vi "DW2BA(glue).vi"(10 "DW01":i16, 11 "DW00":i16) -> (2 "秒數":dbl)   [LabVIEW 2019]
panel:
  out "翻轉後接起再翻轉":u32
  out "翻轉後接起":u32
  out "無翻轉接起後翻轉":u32
  out "無翻轉直接接起來":i32
  out "翻轉後接起再翻轉":bool[](array[boolean])
  out "無翻轉接起後翻轉":bool[](array[boolean])
  out "翻轉後接起":bool[](array[boolean])
  out "無翻轉直接接起來":bool[](array[boolean])
  out "DW01":bool[](array[boolean])
  out "DW00":bool[](array[boolean])
  # "一共有八種可能:\n這邊是DW01+DW00\n另一種是DW00+DW01"
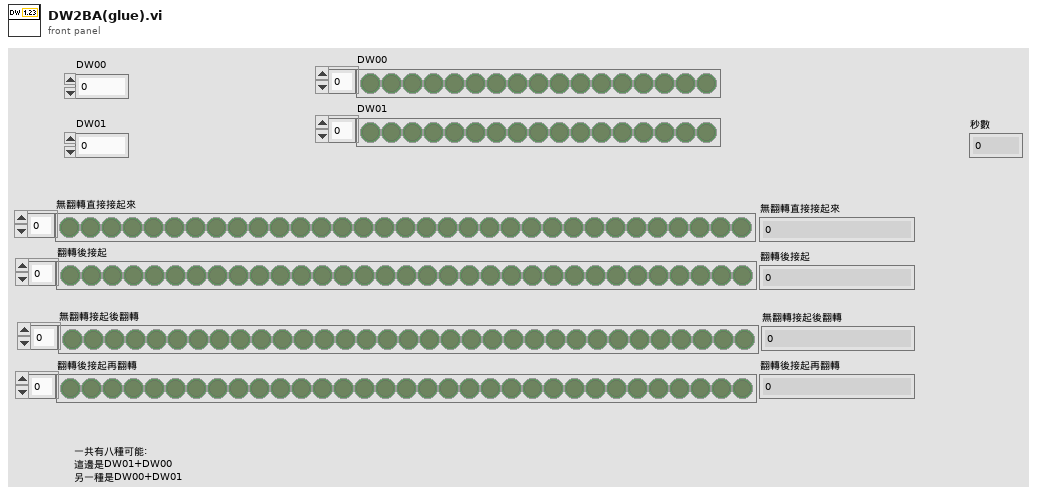
[diagram p1: front panel]
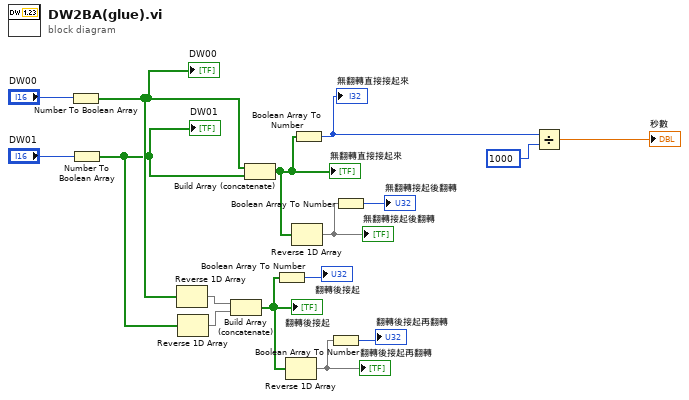
[diagram p0: block diagram]
diagram:
  n1 = Number To Boolean Array(number="DW00") -> (Boolean array=w14:bool[])
  "DW00" <- w14
  n2 = Number To Boolean Array(number="DW01") -> (Boolean array=w13:bool[])
  "DW01" <- w13
  n3 = Reverse 1D Array(array=w14) -> (reversed array=w12:bool[])
  n4 = Reverse 1D Array(array=w13) -> (reversed array=w11:bool[])
  n5 = Build Array (concatenate)(w12, w11) -> (w7:bool[])
  "翻轉後接起" <- w7
  n6 = Build Array (concatenate)(w14, w13) -> (w10:bool[])
  "無翻轉直接接起來" <- w10
  n7 = Boolean Array To Number(Boolean array=w7) -> (number=→"翻轉後接起":u32)
  n8 = Reverse 1D Array(array=w7) -> (reversed array=w5:bool[])
  "翻轉後接起再翻轉" <- w5
  n9 = Reverse 1D Array(array=w10) -> (reversed array=w9:bool[])
  "無翻轉接起後翻轉" <- w9
  n10 = Boolean Array To Number(Boolean array=w10) -> (number=w3:u32)
  "無翻轉直接接起來" <- w3
  n11 = Boolean Array To Number(Boolean array=w5) -> (number=→"翻轉後接起再翻轉":u32)
  n12 = Boolean Array To Number(Boolean array=w9) -> (number=→"無翻轉接起後翻轉":u32)
  n13 = Divide(x=w3, y=u32 1000) -> (x/y=→"秒數":dbl)
